vi "FrameToHeadingPose.vi"(11 "Posture In":dbl[](array[numeric])) -> (0 "Robot Vector":cluster{"Array":dbl[], "Array":dbl[]}, 1 "y":dbl, 2 "x":dbl, 3 "Heading Frame":cluster{"X":sgl, "Y":sgl, "theta":dbl})   [LabVIEW 2016]
uses:
  <vilib>/Analysis/coordinate.llb/Angle Units.ctl
  <vilib>/Analysis/coordinate.llb/Angle Range (Degree).ctl
  <vilib>/Analysis/coordinate.llb/Wrap Angle (scalar).vi
  <vilib>/Analysis/NI_AAL_Angle.lvlib
panel:
  in  "State in":cluster{"X":sgl, "Y":sgl, "theta":dbl}
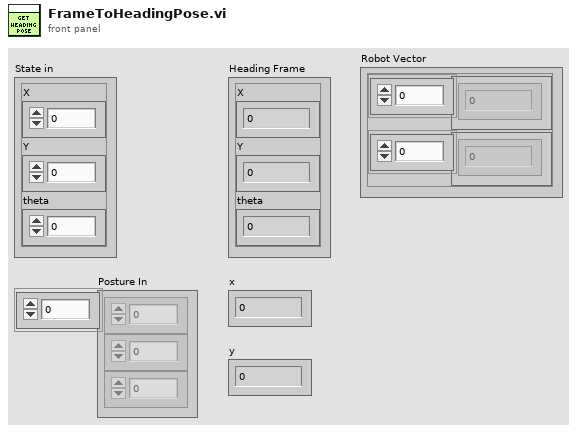
[diagram p1: front panel]
types:
  T1 = typedef "NI_AAL_Angle.lvlib/Angle Range (Degree).ctl" = u16
  T2 = typedef "NI_AAL_Angle.lvlib/Angle Units.ctl" = i32
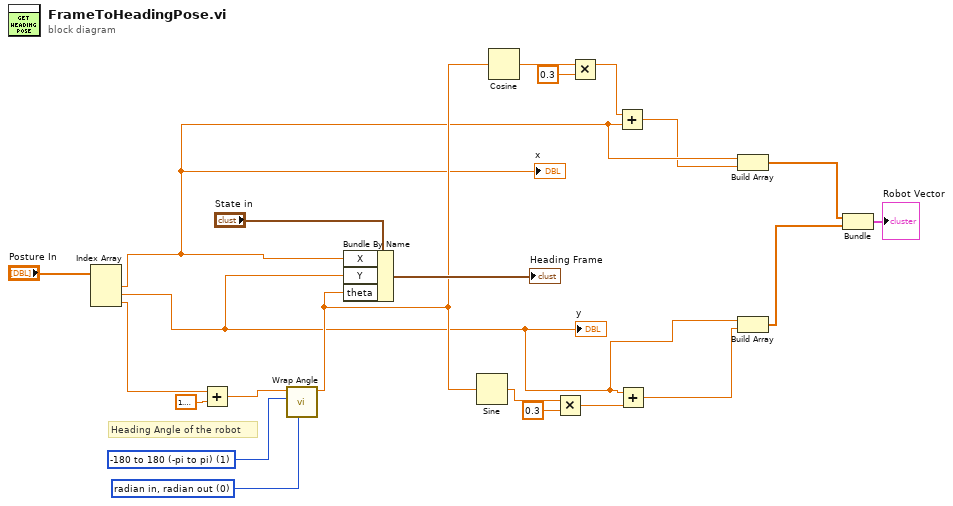
[diagram p0: block diagram]
diagram:
  w16 = T1 1 items=["none", "-180 to 180 (-pi to pi)", "0 to 360 (0 to 2pi)"] ("angle range")
  w17 = T2 0 items=["radian in, radian out", "radian in, degree out", "degree in, degree out", "degree in, radian out"] ("angle units")
  # "Heading Angle of the robot"
  n1 = Index Array(array="Posture In") -> (element #1=w7:dbl, element #2=w4:dbl, element #3=w20:dbl)  [unwired: 3 in]
  "y" <- w4
  "x" <- w7
  n2 = Add(x=w20, y=1.5707963267948966) -> (x+y=w15:dbl)
  n3 = call-poly <vilib>:"Wrap Angle.vi"("angle units"=w17, "angle range"=w16, "angle in"=w15) -> ("angle out"=w13:dbl)  [unwired: 7 in, 1 out]
  n4 = Bundle By Name(cluster="State in", "X"=w7, "Y"=w4, "theta"=w13) -> (→"Heading Frame":cluster{"X":sgl, "Y":sgl, "theta":dbl})
  n5 = Sine(x=w13) -> (sin(x)=w10:dbl)
  n6 = Cosine(x=w13) -> (cos(x)=w14:dbl)
  n7 = Multiply(x=w10, y=0.3) -> (x*y=w8:dbl)
  n8 = Multiply(x=w14, y=0.3) -> (x*y=w12:dbl)
  n9 = Add(x=w12, y=w7) -> (x+y=w6:dbl)
  n10 = Add(x=w4, y=w8) -> (x+y=w5:dbl)
  n11 = Build Array(w7, w6) -> (w3:dbl[])
  n12 = Build Array(w4, w5) -> (w2:dbl[])
  n13 = Bundle(w3, w2) -> (→"Robot Vector":cluster{dbl[], dbl[]})  [unwired: 1 in]
